vi "ProdaNG.Tree.Edit.vi"(6 "reason":string, 7 "TestStepsTree":refnum<vi>, 8 "error in (no error)":errorcluster, 9 "Selected elements values":T1[](array[typedef]), 10 "Selected elements":T2[](array[typedef]), 11 "dbHandleIn":i32) -> (0 "error out":errorcluster, 3 "dbHandle":i32)   [LabVIEW 2016]
uses:
  ProdaNG.Tree.Fglb.Data.ctl
  ProdaNG.Tree.Fglb.Element.ctl
  ProdaNG.Tree.Fglb.Value.ctl
  ProdaNG.Configurator.Glb.vi
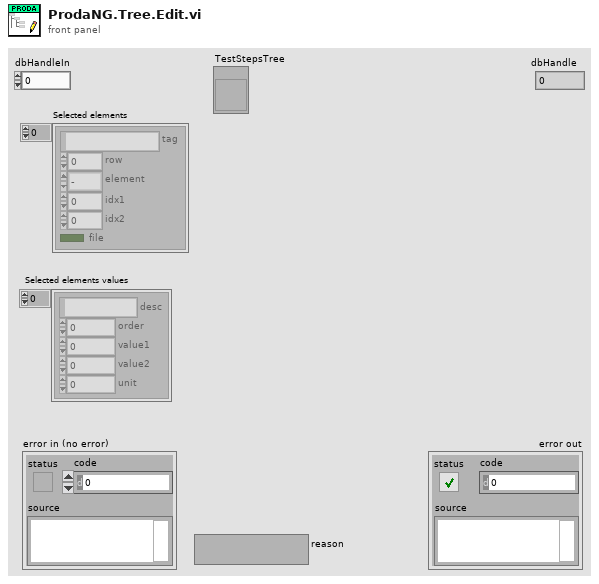
[diagram p1: front panel]
types:
  T1 = typedef "ProdaNG.Tree.Fglb.Value.ctl" = cluster{"desc":string, "order":i32, "value1":dbl, "value2":dbl, "unit":i32}
  T2 = typedef "ProdaNG.Tree.Fglb.Data.ctl" = cluster{"tag":string, "row":i32, "element":T3, "idx1":i32, "idx2":i32, "file":bool}
  T3 = typedef "ProdaNG.Tree.Fglb.Element.ctl" = enum16{"-", "PP", "TS", "TP", "TV"}
  T4 = typedef "ProdaNG.ProcessStepParam.ctl" = cluster{"i_id":i32, "processStepId":i32, "unitId":i32, "contentId":string, "previewId":string, "value":dbl, "valueText":string, "paramSequence":i32, "history":i32, "mdReason":string, "mdUser":string, "mdTime":string, "description":string}
  T5 = typedef "ProdaNG.TestStep.ctl" = cluster{"i_id":i32, "processStepId":i32, "testSequence":i32, "testOrder":i32, "mdReason":string, "mdUser":string, "mdTime":string, "description":string}
  T6 = typedef "ProdaNG.TestStepParam.ctl" = cluster{"i_id":i32, "testStepId":i32, "unitId":i32, "contentId":string, "previewId":string, "value":dbl, "valueText":string, "paramSequence":i32, "history":i32, "mdReason":string, "mdUser":string, "mdTime":string, "description":string}
  T7 = typedef "ProdaNG.TestValue.ctl" = cluster{"i_id":i32, "testStepId":i32, "releaseId":i32, "unitId":i32, "contentId":string, "previewId":string, "maximum":dbl, "minimum":dbl, "valueText":string, "testValueSequence":i32, "history":i32, "mdReason":string, "mdUser":string, "mdTime":string, "description":string}
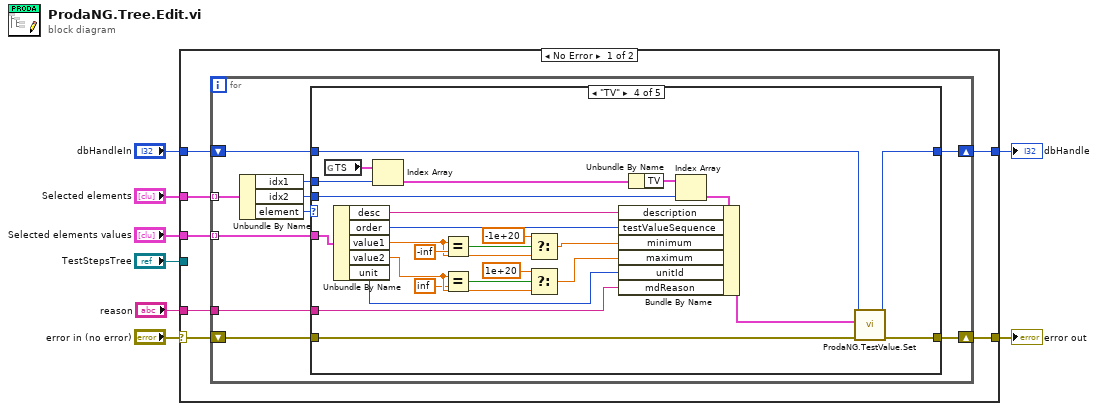
[diagram p0: block diagram]
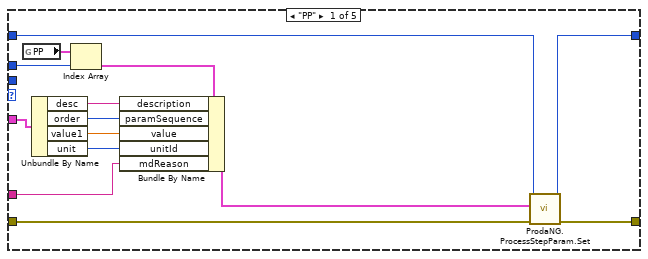
[diagram p2: hidden frame]
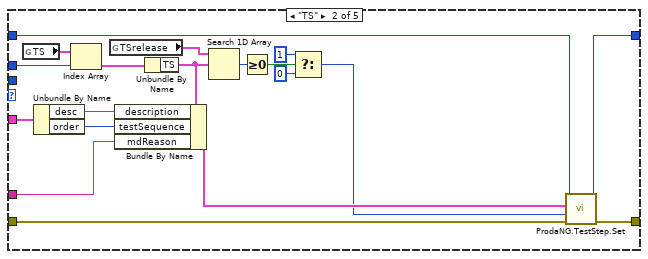
[diagram p3: hidden frame]
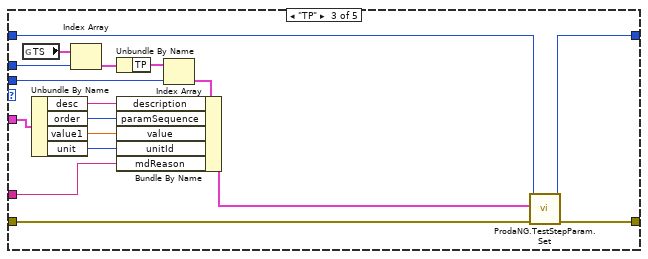
[diagram p4: hidden frame]
diagram:
  n1 = case shown="No Error" "error in (no error)" {
    selector: "error in (no error)" -> [w11 w105]
    tunnel: "TestStepsTree" -> [_ _]
    tunnel: [w15 w105] -> w8
    tunnel: "dbHandleIn" -> [w14 w104]
    tunnel: [w13 w104] -> w4
    tunnel: "Selected elements" -> [w12 _]
    tunnel: "Selected elements values" -> [w10 _]
    tunnel: "reason" -> [w9 _]
    frame No Error {
      n2 = for {
        shift-right: [w23] -> w15
        shift-left: w11 -> [w19]
        shift-right: [w21] -> w13
        shift-left: w14 -> [w22]
        tunnel: w12 -> [w20] mode=indexing
        tunnel: w10 -> [w17] mode=indexing
        tunnel: w9 -> [w16]
        n3 = Unbundle By Name(w20) -> ("idx1"=w24:i32, "idx2"=w18:i32, "element"=w25:T3)
        n4 = case shown="\"TV\"" w25 {
          tunnel: w24 -> [w39 w58 w75 w101 _]
          tunnel: w19 -> [w34 w56 w70 w96 w103]
          tunnel: [w37 w55 w73 w99 w103] -> w23
          tunnel: w22 -> [w36 w54 w72 w98 w102]
          tunnel: [w35 w53 w71 w97 w102] -> w21
          tunnel: w18 -> [_ _ w62 w90 _]
          tunnel: w17 -> [w32 w50 w69 w95 _]
          tunnel: w16 -> [w27 w49 w60 w83 _]
          frame "PP" {
            n5 = global read "ProdaNG.Configurator.Glb.vi" "PP"() -> (w38:T4[])
            n6 = Unbundle By Name(w32) -> ("desc"=w31:string, "order"=w30:i32, "value1"=w29:dbl, "unit"=w26:i32)
            n7 = Index Array(array=w38, index=w39) -> (element=w33:T4)
            n8 = Bundle By Name(cluster=w33, "description"=w31, "paramSequence"=w30, "value"=w29, "unitId"=w26, "mdReason"=w27) -> (w28:T4)
            n9 = call "ProdaNG.ProcessStepParam.Set.vi"("error in (no error)"=w34, "ProcessStepParam"=w28, "dbHandleIn"=w36) -> ("error out"=w37:errorcluster, "dbHandle"=w35:i32)  [unwired: 6 in, 1 out]
          }
          frame "TS" {
            n10 = global read "ProdaNG.Configurator.Glb.vi" "TS"() -> (w57:cluster{"TS":T5, "TP":T6[], "TV":T7[]}[])
            n11 = Unbundle By Name(w50) -> ("desc"=w52:string, "order"=w51:i32)
            n12 = Index Array(array=w57, index=w58) -> (element=w47:cluster{"TS":T5, "TP":T6[], "TV":T7[]})
            n13 = global read "ProdaNG.Configurator.Glb.vi" "TSrelease"() -> (w46:T5[])
            n14 = Unbundle By Name(w47) -> ("TS"=w45:T5)
            n15 = Bundle By Name(cluster=w45, "description"=w52, "testSequence"=w51, "mdReason"=w49) -> (w48:T5)
            n16 = Search 1D Array(1D array=w46, element=w45) -> (index of element=w44:i32)  [unwired: 1 in]
            n17 = Greater Or Equal To 0?(x=w44) -> (x >= 0?=w43:bool)
            n18 = Select(t=1, s=w43, f=0) -> (s? t:f=w40:i32)
            n19 = call "ProdaNG.TestStep.Set.vi"("error in (no error)"=w56, "ReleaseId"=w40, "TestStep"=w48, "dbHandleIn"=w54) -> ("error out"=w55:errorcluster, "dbHandle"=w53:i32)  [unwired: 5 in, 1 out]
          }
          frame "TP" {
            n20 = global read "ProdaNG.Configurator.Glb.vi" "TS"() -> (w74:cluster{"TS":T5, "TP":T6[], "TV":T7[]}[])
            n21 = Unbundle By Name(w69) -> ("desc"=w68:string, "order"=w67:i32, "value1"=w66:dbl, "unit"=w59:i32)
            n22 = Index Array(array=w74, index=w75) -> (element=w64:cluster{"TS":T5, "TP":T6[], "TV":T7[]})
            n23 = Unbundle By Name(w64) -> ("TP"=w63:T6[])
            n24 = Index Array(array=w63, index=w62) -> (element=w61:T6)
            n25 = Bundle By Name(cluster=w61, "description"=w68, "paramSequence"=w67, "value"=w66, "unitId"=w59, "mdReason"=w60) -> (w65:T6)
            n26 = call "ProdaNG.TestStepParam.Set.vi"("error in (no error)"=w70, "TestStepParam"=w65, "dbHandleIn"=w72) -> ("error out"=w73:errorcluster, "dbHandle"=w71:i32)  [unwired: 6 in, 1 out]
          }
          frame "TV" {
            n27 = global read "ProdaNG.Configurator.Glb.vi" "TS"() -> (w100:cluster{"TS":T5, "TP":T6[], "TV":T7[]}[])
            n28 = Unbundle By Name(w95) -> ("desc"=w94:string, "order"=w93:i32, "value1"=w86:dbl, "value2"=w79:dbl, "unit"=w76:i32)
            n29 = Index Array(array=w100, index=w101) -> (element=w92:cluster{"TS":T5, "TP":T6[], "TV":T7[]})
            n30 = Equal?(x=w86, y=-inf) -> (x = y?=w85:bool)
            n31 = Equal?(x=w79, y=inf) -> (x = y?=w80:bool)
            n32 = Select(t=-1e+20, s=w85, f=w86) -> (s? t:f=w82:dbl)
            n33 = Select(t=1e+20, s=w80, f=w79) -> (s? t:f=w77:dbl)
            n34 = Unbundle By Name(w92) -> ("TV"=w91:T7[])
            n35 = Index Array(array=w91, index=w90) -> (element=w89:T7)
            n36 = Bundle By Name(cluster=w89, "description"=w94, "testValueSequence"=w93, "minimum"=w82, "maximum"=w77, "unitId"=w76, "mdReason"=w83) -> (w88:T7)
            n37 = call "ProdaNG.TestValue.Set.vi"("error in (no error)"=w96, "TestValue"=w88, "dbHandleIn"=w98) -> ("error out"=w99:errorcluster, "dbHandle"=w97:i32)  [unwired: 6 in, 1 out]
          }
          frame Default {
          }
        }
      }
    }
    frame Error {
    }
  }
  "error out" <- w8
  "dbHandle" <- w4
